vi "Write Element of Cubes.vi"(8 "error in (no error)":errorcluster, 9 "Cube":refnum<class "Cube.lvclass">, 10 "index":i32, 11 "Cubes in":refnum<class "Cubes.lvclass">) -> (0 "error out":errorcluster, 3 "Cubes out":refnum<class "Cubes.lvclass">)   [LabVIEW 2019, in "22.lvlib" / "Cubes.lvclass"]
uses:
  Cubes.lvclass
  Cube/Cube.lvclass
  Cubes.lvclass/Cubes.ctl
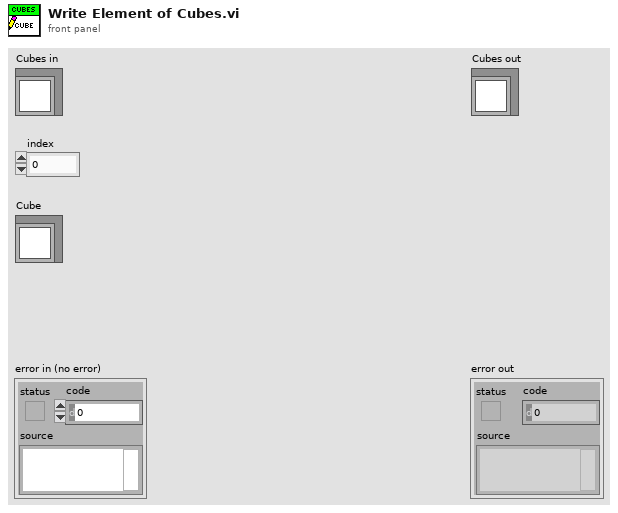
[diagram p1: front panel]
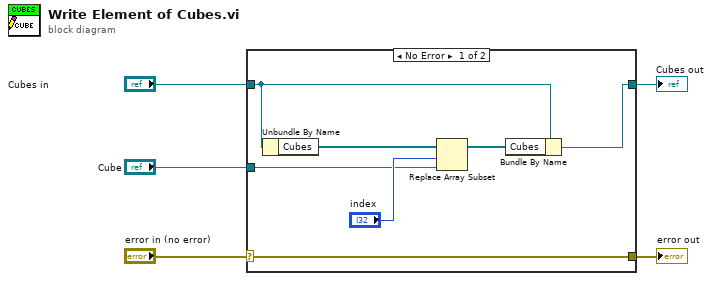
[diagram p0: block diagram]
diagram:
  n1 = case shown="No Error" "error in (no error)" {
    selector: "error in (no error)" -> [w12 w13]
    tunnel: [w12 w13] -> w4
    tunnel: [w11 w14] -> w2
    tunnel: "Cubes in" -> [w10 w14]
    tunnel: "Cube" -> [w6 _]
    frame No Error {
      n2 = Unbundle By Name(w10) -> ("Cubes"=w9:refnum<class "Cube.lvclass">[])
      n3 = Replace Array Subset(array=w9, new element=w6, index="index") -> (w8:refnum<class "Cube.lvclass">[])
      n4 = Bundle By Name(cluster=w10, "Cubes"=w8) -> (w11:refnum<class "Cubes.lvclass">)
    }
    frame Error {
    }
  }
  "error out" <- w4
  "Cubes out" <- w2
